vi "WT1800 Bundle Function Names.vi"(0 "Element Group":i32, 5 "Number of Elements":i32, 7 "Number of Functions":i32, 9 "Array in":string[](array[string]), 11 "Function":string[](array[string])) -> (4 "Array out":T1(array[cluster]))   [LabVIEW 2015]
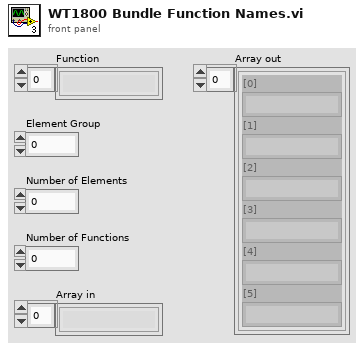
[diagram p1: front panel]
types:
  T1 = cluster{"[0]":string, "[1]":string, "[2]":string, "[3]":string, "[4]":string, "[5]":string}[]
  T2 = cluster{"[0]":string, "[1]":string, "[2]":string, "[3]":string, "[4]":string, "[5]":string}
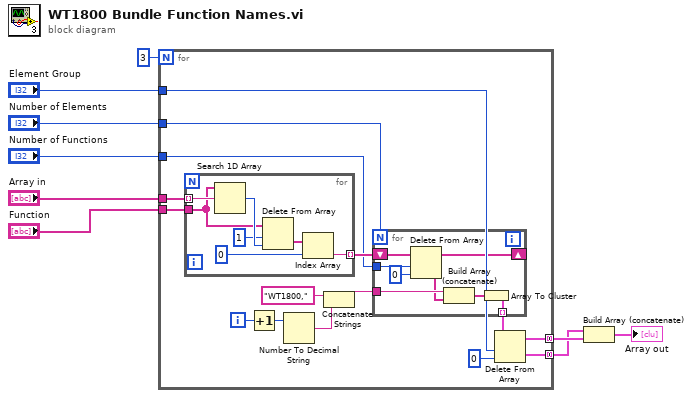
[diagram p0: block diagram]
diagram:
  n1 = for {
    N: 3 -> [_]
    tunnel: "Array in" -> [w23]
    tunnel: "Function" -> [w22]
    tunnel: "Number of Functions" -> [w13]
    tunnel: "Number of Elements" -> [w21]
    tunnel: [w11] -> w6 mode=concatenating
    tunnel: [w12] -> w5 mode=concatenating
    tunnel: "Element Group" -> [w10]
    i -> [w18]
    n2 = for {
      tunnel: w22 -> [w33]
      tunnel: w23 -> [w39] mode=indexing
      tunnel: [w34] -> w15 mode=indexing
      n3 = Search 1D Array(1D array=w33, element=w39) -> (index of element=w38:i32)  [unwired: 1 in]
      n4 = Delete From Array(array=w33, length=1, index=w38) -> (deleted portion=w36:string[])  [unwired: 1 out]
      n5 = Index Array(array=w36, index=0) -> (element=w34:string)
    }
    n6 = Increment(x=w18) -> (x+1=w17:i32)
    n7 = Number To Decimal String(number=w17) -> (decimal integer string=w16:string)  [unwired: 1 in]
    n8 = Concatenate Strings("WT1800," ("string"), w16) -> (w14:string)
    n9 = for {
      N: w21 -> [_]
      shift-right: [w31] -> _
      shift-left: w15 -> [w32]
      tunnel: w13 -> [w30]
      tunnel: [w28] -> w24 mode=indexing
      tunnel: w14 -> [w27]
      n10 = Delete From Array(array=w32, length=w30, index=0) -> (deleted portion=w26:string[], array with subset deleted=w31:string[])
      n11 = Build Array (concatenate)(w27, w26) -> (w25:string[])
      n12 = Array To Cluster(array=w25) -> (cluster=w28:T2)
    }
    n13 = Delete From Array(array=w24, length=w10, index=0) -> (deleted portion=w12:T1, array with subset deleted=w11:T1)
  }
  n14 = Build Array (concatenate)(w5, w6) -> (→"Array out":T1)
